vi "PID motor Sharp.vi"() -> ()   [LabVIEW 2012]
uses:
  <vilib>/Analysis/baseanly.llb/Mean (DBL).vi
  <vilib>/Analysis/NI_AALBase.lvlib
panel:
  in  "Cutoff Frequency":dbl=10.0 format="%0.4f"
  out "error":dbl(slide) scale=-5.0..5.0
  out "error":dbl
  out "Td 3":dbl=0.3305785123966942
  out "kp 3":dbl=0.24793388429752067
  out "Td 2":dbl=0.43388429752066116
  in  "Ti":dbl(slide)=0.4132231404958678 scale=0.0..5.0
  in  "Td":dbl(slide)=0.3305785123966942 scale=0.0..5.0
  in  "Kp":dbl(slide)=0.3925619834710744 scale=0.0..5.0
  out "Respuesta del Sistema":dynamicdata(graph)
  in  "Tiempo de muestreo":dbl=0.019
  in  "OFF":bool
  # "VARIABLES DEL CONTROL PID"
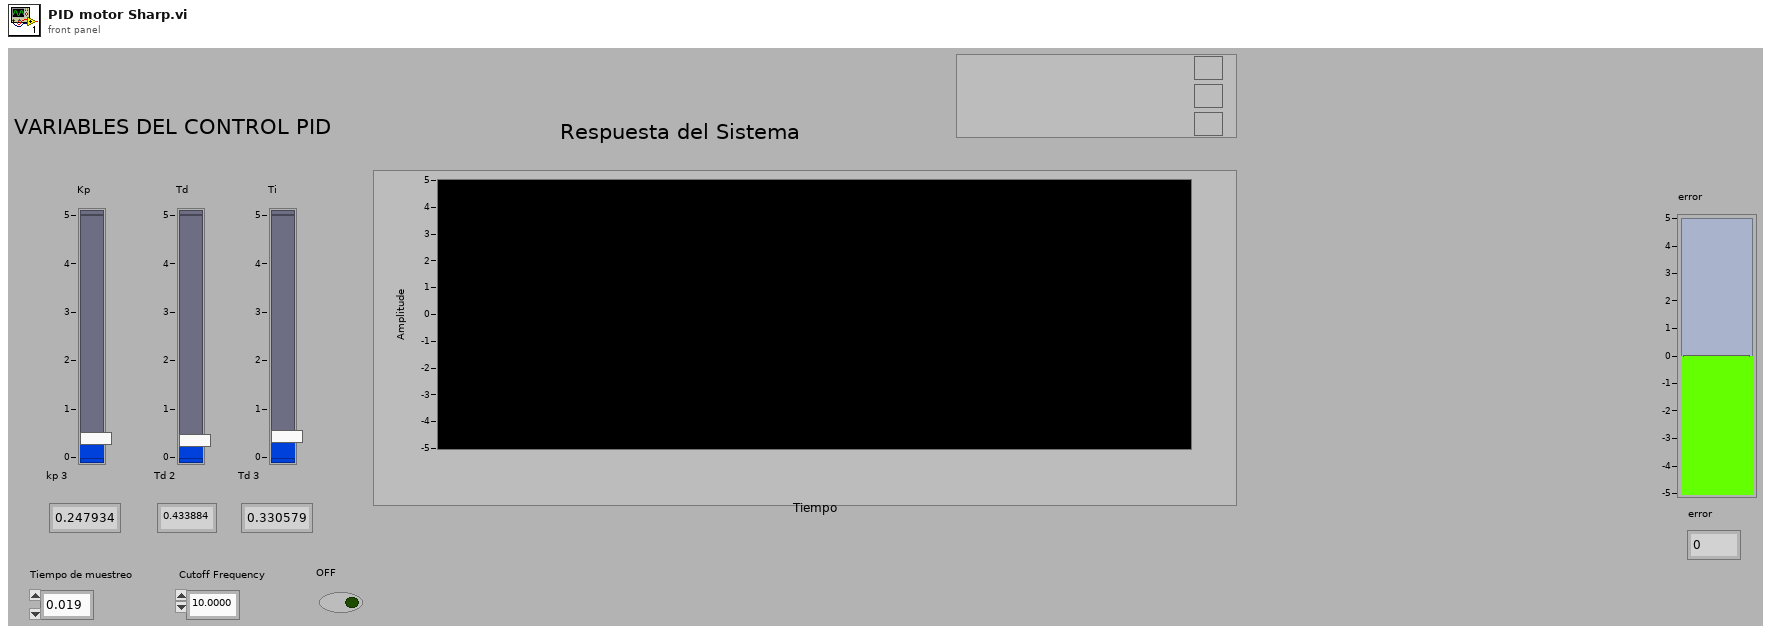
[diagram p1: front panel]
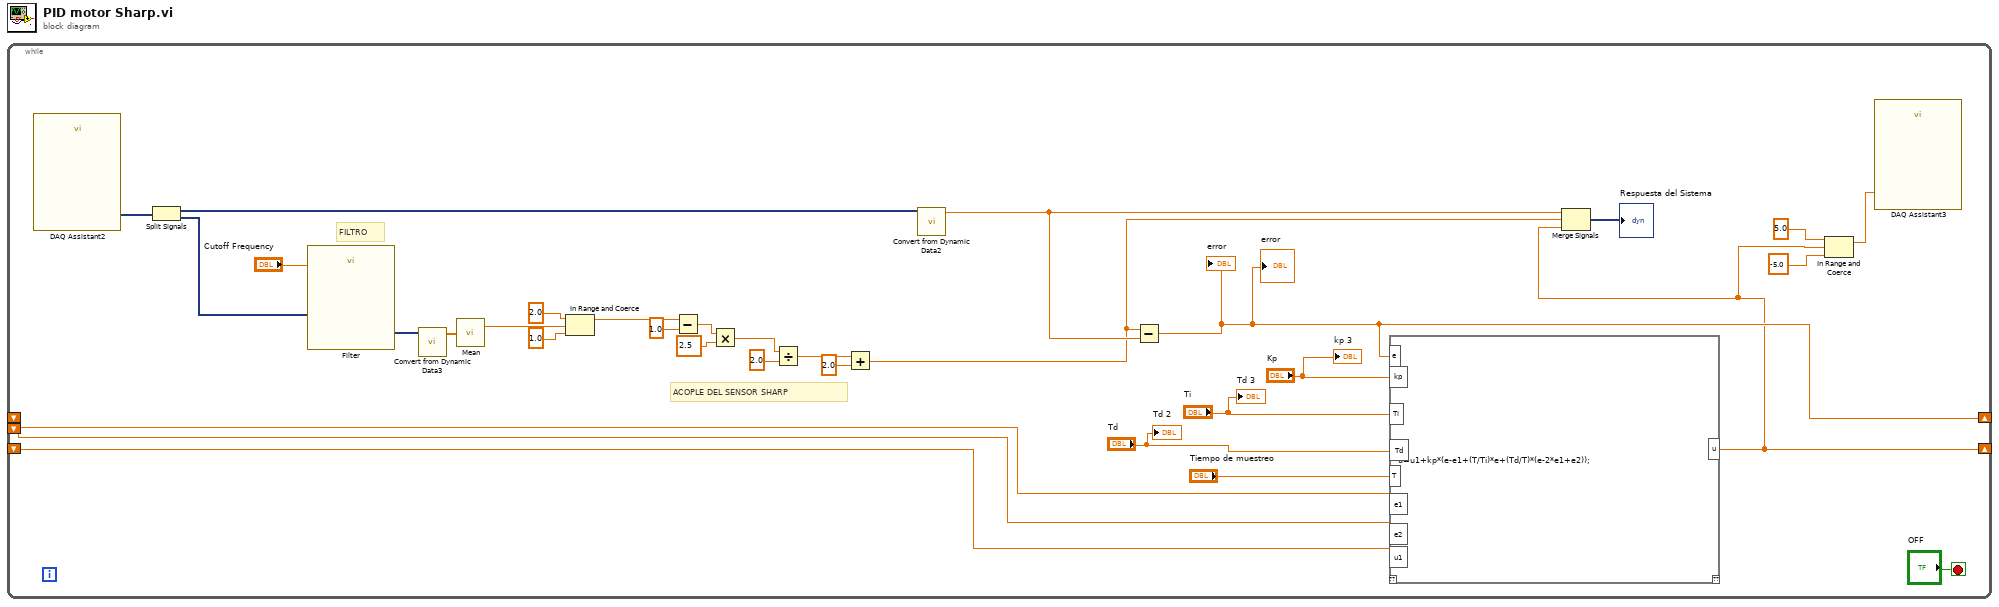
[diagram p0: block diagram]
diagram:
  n1 = while {
    shift-right: [w20] -> _
    shift-left: _ -> [w33]
    shift-right: [w21] -> _
    shift-left: _ -> [w32]
    shift-left: _ -> [w31]
    stop <- "OFF" stop-if-true
    # "FILTRO"
    # "ACOPLE DEL SENSOR SHARP"
    n2 = call "DAQ Assistant2"() -> ("data"=w18:dynamicdata)  [unwired: 17 in, 2 out]
    n3 = Split Signals(w18) -> (w17:dynamicdata, w2:dynamicdata)  [unwired: 2 in]
    n4 = call "Filter"("Lower Cut-Off"="Cutoff Frequency", "Signal"=w2) -> ("Filtered Signal"=w14:dynamicdata)  [unwired: 8 in, 1 out]
    n5 = call "Convert from Dynamic Data3"("Dynamic Data Type"=w14) -> ("Array"=w15:dbl[])  [unwired: 3 in]
    n6 = call-poly <vilib>:"Mean.vi"("X"=w15) -> ("mean"=w3:dbl)  [unwired: 1 out]
    n7 = In Range and Coerce(upper limit=2.0, x=w3, lower limit=1.0) -> (coerced(x)=w1:dbl)  [unwired: 1 out]
    n8 = Subtract(x=w1, y=1.0) -> (x-y=w7:dbl)
    n9 = Multiply(x=w7, y=2.5) -> (x*y=w9:dbl)
    n10 = Divide(x=w9, y=2.0) -> (x/y=w5:dbl)
    n11 = Add(x=w5, y=2.0) -> (x+y=w4:dbl)
    n12 = call "Convert from Dynamic Data2"("Dynamic Data Type"=w17) -> ("Scalar"=w19:dbl)  [unwired: 3 in]
    n13 = Subtract(x=w4, y=w19) -> (x-y=w21:dbl)
    "error" <- w21
    "error" <- w21
    n14 = script code="u=u1+kp*(e-e1+(T/Ti)*e+(Td/T)*(e-2*e1+e2));"("kp"="Kp", "Ti"="Ti", "Td"="Td", "T"="Tiempo de muestreo", "e2"=w31, "e"=w21, "u1"=w33, "e1"=w32) -> ("u"=w20:dbl)  [unwired: 1 in, 1 out]
    n15 = Merge Signals(w19, w4, w20) -> (→"Respuesta del Sistema":dynamicdata)
    n16 = In Range and Coerce(upper limit=5.0, x=w20, lower limit=-5.0) -> (coerced(x)=w25:dbl)  [unwired: 1 out]
    n17 = call "DAQ Assistant3"("data"=w25) -> ()  [unwired: 17 in, 2 out]
    "Td 2" <- "Td"
    "kp 3" <- "Kp"
    "Td 3" <- "Ti"
  }
